vi "Set_Save_Test_Data_Result.vi"(10 "Result Arry":string[](array[string]), 11 "测试数据 2":refnum<vi>) -> (3 "测试数据 3":refnum<vi>)   [LabVIEW 2018]
uses:
  <vilib>/Utility/miscctls.llb/LVRowAndColumnTypeDef.ctl
panel:
  in  "测试数据":i32(listbox)
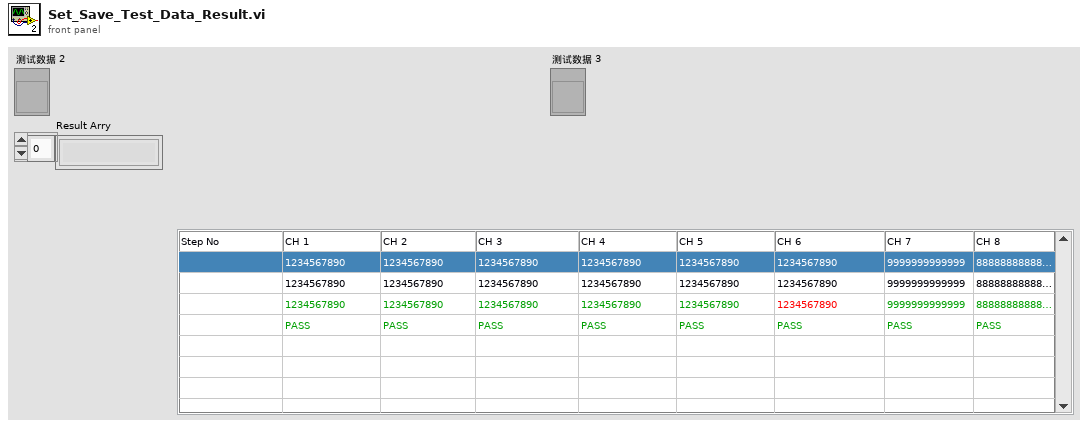
[diagram p1: front panel]
types:
  T1 = typedef "LVRowAndColumnTypeDef.ctl" = cluster{"Row":i32, "Column":i32}
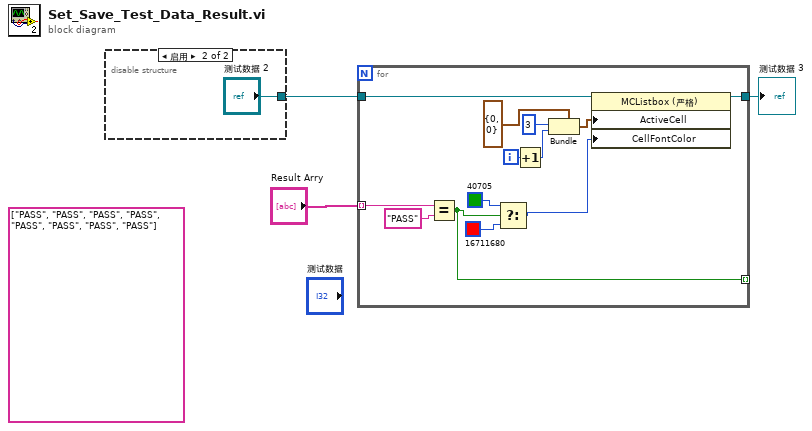
[diagram p0: block diagram]
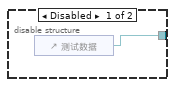
[diagram p2: hidden frame]
diagram:
  (unwired) string[] ["PASS", "PASS", "PASS", "PASS", "PASS", "PASS", "PASS", "PASS"]
  n1 = disable-structure shown="启用" {
    disable-tunnel: [w4 "测试数据 2"] -> w3
    frame Disabled {
      n2 = control-ref of="测试数据"() -> (w4:refnum<vi>)
    }
    frame Enabled {
    }
  }
  n3 = for {
    tunnel: w3 -> [w18]
    tunnel: "Result Arry" -> [w15] mode=indexing
    tunnel: [w13] -> w2
    tunnel: [w6] -> _ mode=indexing
    i -> [w11]
    n4 = Equal?(x=w15, y="PASS") -> (x = y?=w6:bool)
    n5 = Select(t=u32 40705, s=w6, f=u32 16711680) -> (s? t:f=w7:u32)
    n6 = Increment(x=w11) -> (x+1=w10:i32)
    n7 = Bundle(cluster=T1 {"Row"=0, "Column"=0} ("活动单元格:活动单元格"), "Row"=3 ("Column"), "Column"=w10) -> (w16:T1)
    n8 = property class="MCListbox (严格)"(reference=w18, "ActiveCell"=w16, "CellFontColor"=w7) -> (reference out=w13:refnum<vi>)  [unwired: 1 in, 1 out]
  }
  "测试数据 3" <- w2
